vi "Check for 'set' errors.vi"(8 "error in (no error)":errorcluster, 10 "return value":i32) -> (0 "error out":errorcluster, 2 "return value out":i32)   [LabVIEW 2015]
doc: "Takes the result of a 'set' operation on the wavelength meter and checks for errors."
uses:
  <vilib>/Utility/error.llb/DialogType.ctl
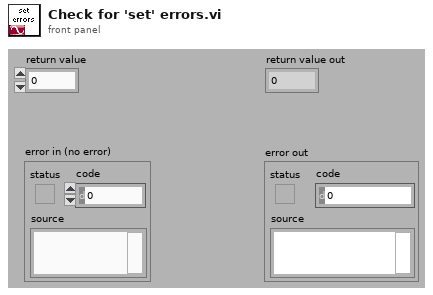
[diagram p1: front panel]
types:
  T1 = typedef "DialogType.ctl" = u16
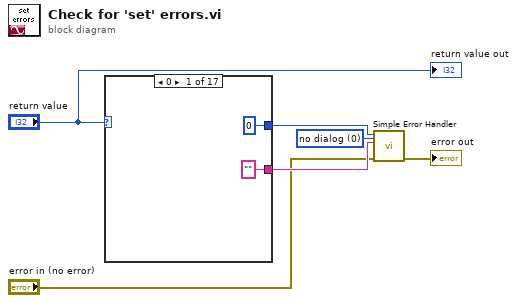
[diagram p0: block diagram]
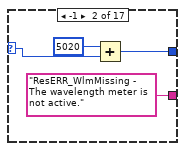
[diagram p2: hidden frame]
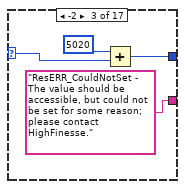
[diagram p3: hidden frame]
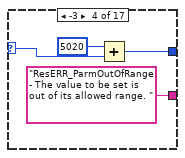
[diagram p4: hidden frame]
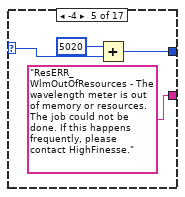
[diagram p5: hidden frame]
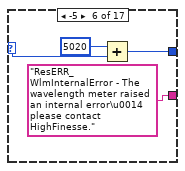
[diagram p6: hidden frame]
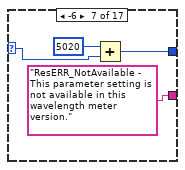
[diagram p7: hidden frame]
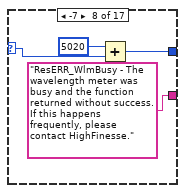
[diagram p8: hidden frame]
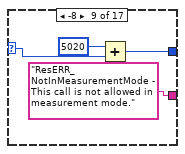
[diagram p9: hidden frame]
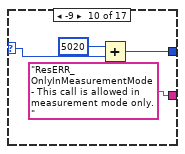
[diagram p10: hidden frame]
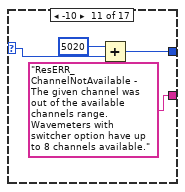
[diagram p11: hidden frame]
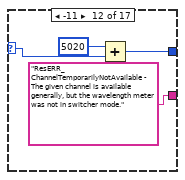
[diagram p12: hidden frame]
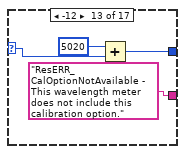
[diagram p13: hidden frame]
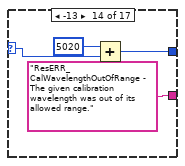
[diagram p14: hidden frame]
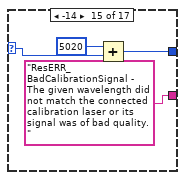
[diagram p15: hidden frame]
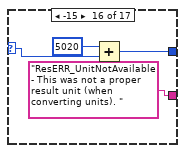
[diagram p16: hidden frame]
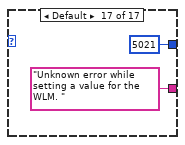
[diagram p17: hidden frame]
diagram:
  w6 = T1 0 items=["no dialog", "OK message", "continue or stop message", "OK message + warnings", "continue/stop + warnings"] ("type of dialog (OK msg:1)")
  n1 = case shown="0" "return value" {
    selector: "return value" -> [_ w10 w14 w18 w22 w26 w29 w33 w38 w42 w46 w50 w54 w57 w61 w66 _]
    tunnel: ["" ("error source (\" \")") "ResERR_WlmMissing - The wavelength meter is not active." ("error source (\" \")") "ResERR_CouldNotSet - The value should be accessible, but could not be set for some reason; please contact HighFinesse." ("error source (\" \")") "ResERR_ParmOutOfRange - The value to be set is out of its allowed range. " ("error source (\" \")") "ResERR_WlmOutOfResources - The wavelength meter is out of memory or resources. The job could not be done. If this happens frequently, please contact HighFinesse." ("error source (\" \")") "ResERR_WlmInternalError - The wavelength meter raised an internal error\u0014 please contact HighFinesse." ("error source (\" \")") "ResERR_NotAvailable - This parameter setting is not available in this wavelength meter version." ("error source (\" \")") "ResERR_WlmBusy - The wavelength meter was busy and the function returned without success. If this happens frequently, please contact HighFinesse." ("error source (\" \")") "ResERR_NotInMeasurementMode - This call is not allowed in measurement mode." ("error source (\" \")") "ResERR_OnlyInMeasurementMode - This call is allowed in measurement mode only." ("error source (\" \")") "ResERR_ChannelNotAvailable - The given channel was out of the available channels range. Wavemeters with switcher option have up to 8 channels available." ("error source (\" \")") "ResERR_ChannelTemporarilyNotAvailable - The given channel is available generally, but the wavelength meter was not in switcher mode." ("error source (\" \")") "ResERR_CalOptionNotAvailable - This wavelength meter does not include this calibration option." ("error source (\" \")") "ResERR_CalWavelengthOutOfRange - The given calibration wavelength was out of its allowed range." ("error source (\" \")") "ResERR_BadCalibrationSignal - The given wavelength did not match the connected calibration laser or its signal was of bad quality." ("error source (\" \")") "ResERR_UnitNotAvailable - This was not a proper result unit (when converting units). " ("error source (\" \")") "Unknown error while setting a value for the WLM. " ("error source (\" \")")] -> w5
    tunnel: [0 w9 w13 w17 w21 w25 w30 w34 w37 w41 w45 w49 w53 w58 w62 w65 5021] -> w2
    frame 0 {
    }
    frame -1 {
      n2 = Add(x=5020, y=w10) -> (x+y=w9:i32)
    }
    frame -2 {
      n3 = Add(x=5020, y=w14) -> (x+y=w13:i32)
    }
    frame -3 {
      n4 = Add(x=5020, y=w18) -> (x+y=w17:i32)
    }
    frame -4 {
      n5 = Add(x=5020, y=w22) -> (x+y=w21:i32)
    }
    frame -5 {
      n6 = Add(x=5020, y=w26) -> (x+y=w25:i32)
    }
    frame -6 {
      n7 = Add(x=5020, y=w29) -> (x+y=w30:i32)
    }
    frame -7 {
      n8 = Add(x=5020, y=w33) -> (x+y=w34:i32)
    }
    frame -8 {
      n9 = Add(x=5020, y=w38) -> (x+y=w37:i32)
    }
    frame -9 {
      n10 = Add(x=5020, y=w42) -> (x+y=w41:i32)
    }
    frame -10 {
      n11 = Add(x=5020, y=w46) -> (x+y=w45:i32)
    }
    frame -11 {
      n12 = Add(x=5020, y=w50) -> (x+y=w49:i32)
    }
    frame -12 {
      n13 = Add(x=5020, y=w54) -> (x+y=w53:i32)
    }
    frame -13 {
      n14 = Add(x=5020, y=w57) -> (x+y=w58:i32)
    }
    frame -14 {
      n15 = Add(x=5020, y=w61) -> (x+y=w62:i32)
    }
    frame -15 {
      n16 = Add(x=5020, y=w66) -> (x+y=w65:i32)
    }
    frame Default {
    }
  }
  n17 = call <vilib>:"Simple Error Handler.vi"("error code (no error:0)"=w2, "error source (\" \")"=w5, "type of dialog (OK msg:1)"=w6, "error in (no error)"="error in (no error)") -> ("error out"=→"error out":errorcluster)  [unwired: 5 out]
  "return value out" <- "return value"
